vi "2_2_PatchCore_Inference(Camera).vi"() -> ()   [LabVIEW 2024]
uses:
  <vilib>/Ngene/DeepLTK Anomaly Detection Addon/DeepLTK_Anomaly_Detection_Addon/API/Controls/NN_Paths.ctl
  <vilib>/Ngene/Deep Learning Toolkit/Toolkit/NN_Data/API/NN_Dims(C,H,W).ctl
  <vilib>/Ngene/Deep Learning Toolkit/Toolkit/NN_Network/Controls/NN_Device.ctl
  subVIs/Visualizer/Controls/Display_Options.ctl
  subVIs/Visualizer/Controls/ROI_Display_Options.ctl
  subVIs/Visualizer/Controls/Heatmap_Display_Options.ctl
  subVIs/Visualizer/Controls/ColorMap.ctl
  <vilib>/Ngene/DeepLTK Anomaly Detection Addon/DeepLTK_Anomaly_Detection_Addon/API/Controls/MinMax.ctl
  subVIs/Camera/Controls/Camera_Settings.ctl
  <vilib>/Ngene/DeepLTK Anomaly Detection Addon/DeepLTK_Anomaly_Detection_Addon/API/Controls/NNPC_Setup.ctl
  <vilib>/vision/driver/IMAQdx.llb/IMAQdx Camera Control Mode.ctl
  <vilib>/vision/driver/IMAQdx.llb/IMAQdx Buffer Number Mode.ctl
  <vilib>/Ngene/DeepLTK Anomaly Detection Addon/DeepLTK_Anomaly_Detection_Addon/API/Controls/Feature_Scorer_Params.ctl
  <vilib>/Ngene/DeepLTK Anomaly Detection Addon/DeepLTK_Anomaly_Detection_Addon/API/Controls/Gaussian_Blur.ctl
  <vilib>/Ngene/DeepLTK Anomaly Detection Addon/DeepLTK_Anomaly_Detection_Addon/API/NNPC_Predict/NNPC_Predict(Single).vi
  <vilib>/Ngene/DeepLTK Anomaly Detection Addon/DeepLTK_Anomaly_Detection_Addon/DeepLTK_Anomaly_Detection_Addon.lvlib
  <vilib>/ptbypt/NI_PtbyPt.lvlib
  <vilib>/vision/driver/NI_Vision_Acquisition_Software.lvlib
  <vilib>/Ngene/Deep Learning Toolkit/Toolkit/Deep_Learning_Toolkit_by_Ngene.lvlib
  <vilib>/Ngene/CuLab - GPU Accelerated Toolkit/Toolkit/CuLab.lvlib
panel:
  in  "Tab Control":enum32{"Config", "Demo"}(tab)=enum."Demo"
  in  "Center_Crop_Size":i32=800
  in  "Device":T1
  in  "Trained_Model_Paths":T2={"CFG"=path "D:/Ngene/Projects_SVN/AD/Projects/2025/2025_04_09_VAD_RT_NIConnect/Models/NNPC_Cards_v2__25_04_09__17_01_43/NNPC_Cards_v2.cfg", "BIN"=path "D:/Ngene/Projects_SVN/AD/Projects/2025/2025_04_09_VAD_RT_NIConnect/Models/NNPC_Cards_v2__25_04_09__17_01_43/NNPC_Cards_v2.bin"}
  in  "Display_Options":T3={"ROI_Options"={"Color"=16711713, "Width"=4, "Drawing Mode"=enum."Frame"}, "Heatmap_Options"={"ColorMap"=enum."Jet", "Alpha"=0.4, "Heatmap Range"={"Min"=6.0, "Max"=-1.0}}, "Has GT?"=FALSE} {"Heatmap_Options"."Heatmap Range"."Min" format="%#_5g"}
  in  "Camera":refnum<k21>="cam5" caption="IMAQdx Session"
  in  "Rel Margin":sgl=0.02
  in  "Camera_Settings":T8={"Camera_Resolution"=270, "Focus"=17, "Exposure"=2, "Gain"=34, "WhiteB."=6457} {"WhiteB." min=2800 max=6500 step=1; "Gain" max=0; "Exposure" min=0 max=8 step=1; "Focus" max=0}
  out "Error Count":i16
  in  "Image_Thrshld":sgl=-1.0 format="%_5g"
  out "Pixel_Score(Max)":sgl=12.824394
  out "Img_Score":sgl=14.272138
  in  "Pixel_Thrshld":sgl=7.0 format="%_5g"
  out "Loop Time":dbl=0.692728653499671 format="%.2ps"
  out "Preproc. Time":dbl=0.014120406500296667 format="%.2ps"
  out "Dims_In":T9={"C"=3, "H"=256, "W"=256}
  in  "Stop":bool
  out "FPS":dbl=1.5954872600149606 format="%_3p"
  out "Inference Time":dbl=0.6267677749997347 format="%_3p"
  out "Device Name":string="sbRIO-9609"
  out "Prediction":bool=TRUE
  out "Anomaly Detection Results":T10(plugin-control)
  # "Unsupervised \nVisual Anomaly Detection"
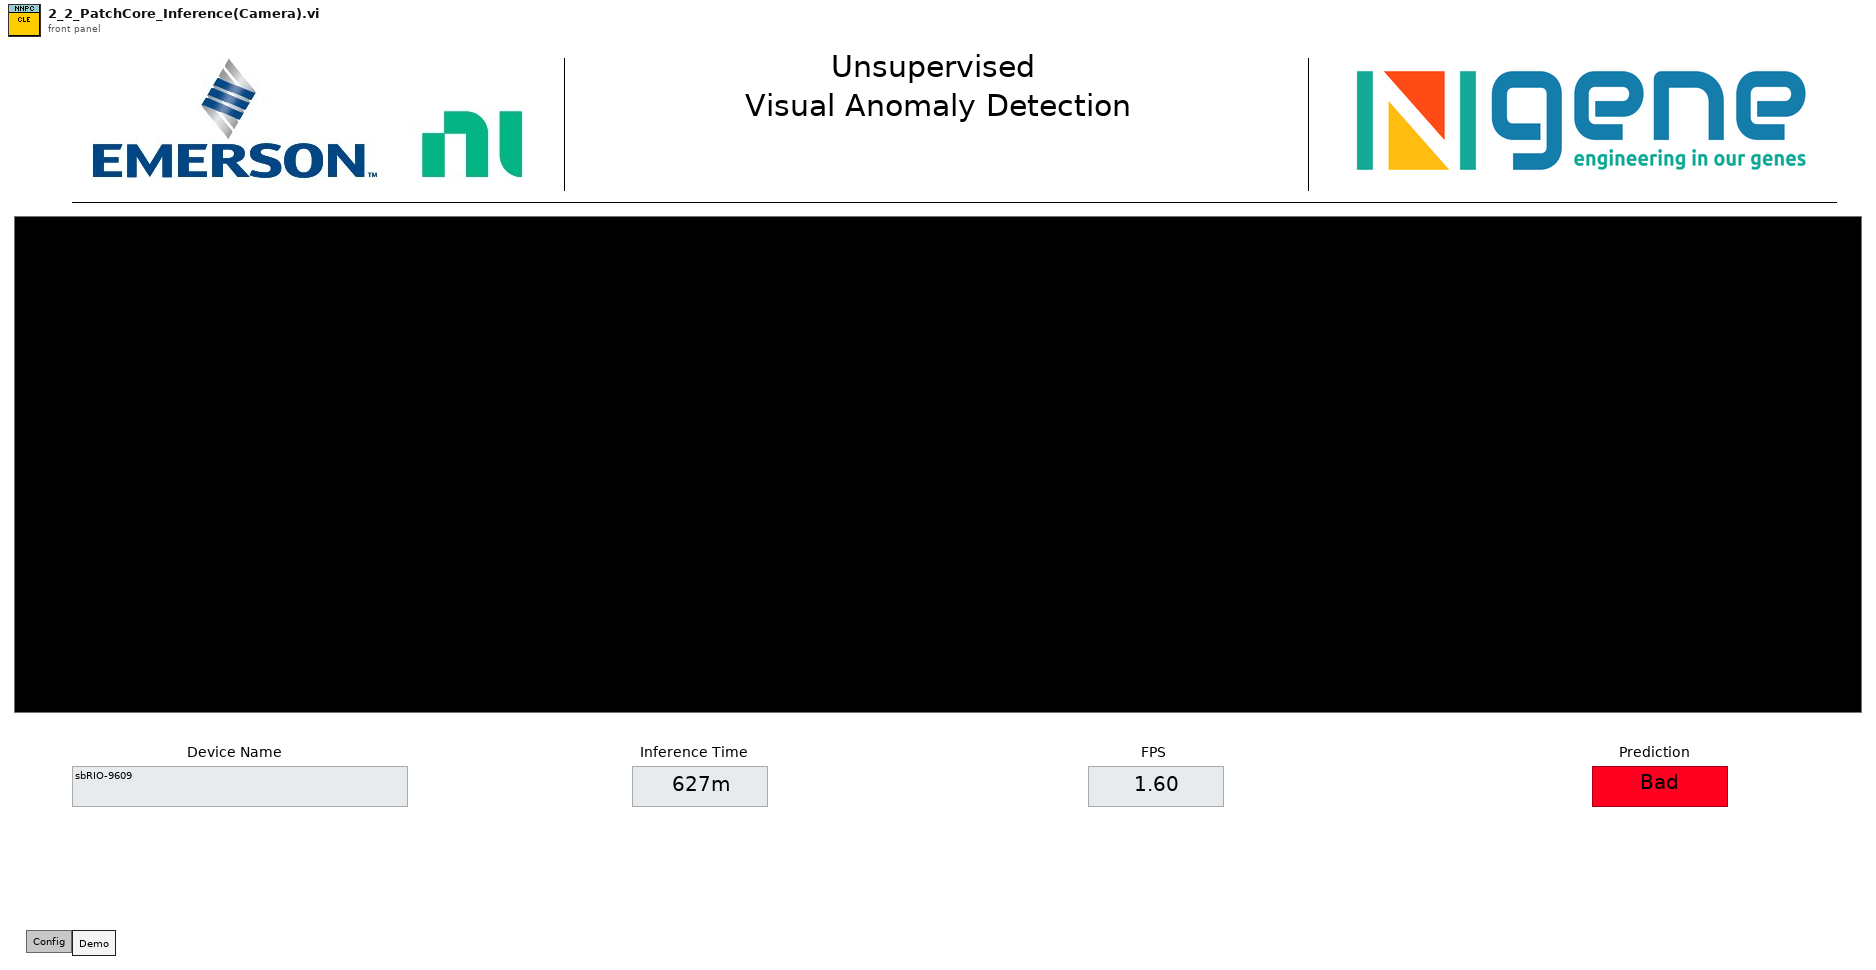
[diagram p1: front panel]
types:
  T1 = typedef "Deep_Learning_Toolkit_by_Ngene.lvlib/NN_Device.ctl" = enum16{"CPU", "GPU"}
  T2 = typedef "DeepLTK_Anomaly_Detection_Addon.lvlib/NN_Paths.ctl" = cluster{"CFG":path, "BIN":path}
  T3 = typedef "Display_Options.ctl" = cluster{"ROI_Options":T4, "Heatmap_Options":T5, "Has GT?":bool}
  T4 = typedef "ROI_Display_Options.ctl" = cluster{"Color":u32, "Width":u32, "Drawing Mode":enum16{"Frame", "Fill"}}
  T5 = typedef "Heatmap_Display_Options.ctl" = cluster{"ColorMap":T6, "Alpha":sgl, "Heatmap Range":T7}
  T6 = typedef "ColorMap.ctl" = enum16{"Jet", "Perula", "Inferno", "Plasma", "Viridis"}
  T7 = typedef "DeepLTK_Anomaly_Detection_Addon.lvlib/MinMax.ctl" = cluster{"Min":sgl, "Max":sgl}
  T8 = typedef "Camera_Settings.ctl" = cluster{"Camera_Resolution":i32, "Focus":u8, "Exposure":i32, "Gain":u32, "WhiteB.":i32}
  T9 = typedef "Deep_Learning_Toolkit_by_Ngene.lvlib/NN_Dims(C,H,W).ctl" = cluster{"C":i32, "H":i32, "W":i32}
  T10 = typedef "IMAQ Image.ctl" = refnum<image>
  T11 = typedef "Image Type" = u32
  T12 = typedef "NI_Vision_Acquisition_Software.lvlib/IMAQdx Camera Control Mode.ctl" = enum32{"Controller", "Listener"}
  T13 = typedef "DeepLTK_Anomaly_Detection_Addon.lvlib/NNPC_Setup.ctl" = cluster{"Input_Dims":T9, "mBatch":i32, "Device":T1, "GPU Id":i32}
  T14 = typedef "IMAQdx.ctl" = refnum<k21>
  T15 = typedef "DeepLTK_Anomaly_Detection_Addon.lvlib/NNPC_Evaluation_Results.ctl" = cluster{"Threshold(Image)":sgl, "Threshold(Pixel)":sgl, "Pixel_Range":cluster{"Min":sgl, "Max":sgl}}
  T16 = typedef "DeepLTK_Anomaly_Detection_Addon.lvlib/NNPC_PreProcessing_Options.ctl" = cluster{"DS_Name":string, "Input_Dims":T9, "Center Crop Size":i32, "Interpolation Type":u32, "Multi-Stage_DownSample?":bool, "Dataset_Stats":T17}
  T17 = typedef "DeepLTK_Anomaly_Detection_Addon.lvlib/NNPC_DS_Stats.ctl" = cluster{"means":T18, "stds":T18}
  T18 = typedef "DeepLTK_Anomaly_Detection_Addon.lvlib/Image_Stats_RGB.ctl" = cluster{"R":sgl, "G":sgl, "B":sgl}
  T19 = typedef "DeepLTK_Anomaly_Detection_Addon.lvlib/NNPC_Instance.ctl" = cluster{"NN out":T20, "MemBank_Data":T35, "Name":string}
  T20 = typedef "Deep_Learning_Toolkit_by_Ngene.lvlib/NN.ctl" = cluster{"Name":string, "No of Layers":i32, "mBatch":i32, "Layers":T21[], "Dimty":T22, "Dims_In":T9, "Dims_Out":T9, "Working_Dir":path, "Train?":bool, "Train_Params":T23, "LR_Update_Policy":T26, "Session Data":T28, "Ground_truth":T29, "NNg_hdls":T30, "NN_Device":T1, "GPU Id":i32, "Labels":string[], "Receptive Field":T31[], "Loss_Type":T32, "Loss_Cfg_Prms":variant, "NNG_WS":T33}
  T21 = typedef "Deep_Learning_Toolkit_by_Ngene.lvlib/NN_Layer_ref.ctl" = refnum<data-value>
  T22 = typedef "Deep_Learning_Toolkit_by_Ngene.lvlib/NN_In_Out_Dim-ty.ctl" = enum8{"In1D_Out1D", "In3D_Out1D", "In3D_Out3D", "In3D_OutBBox"}
  T23 = typedef "Deep_Learning_Toolkit_by_Ngene.lvlib/NN_Train_Params.ctl" = cluster{"Optimizer":T24, "Beta_1":sgl, "Beta_2":sgl, "Weight Decay(L1)":sgl, "Weight Decay(L2)":sgl, "Data_Sampling":T25}
  T24 = typedef "Deep_Learning_Toolkit_by_Ngene.lvlib/NN_Train_Optimizer.ctl" = enum16{"SGD", "Adam", "Adagrad", "Adadelta", "RMSProp", "Nesterov"}
  T25 = typedef "Deep_Learning_Toolkit_by_Ngene.lvlib/NN_Train_Data_Sampling.ctl" = enum16{"Random", "Sequential"}
  T26 = typedef "Deep_Learning_Toolkit_by_Ngene.lvlib/NN_LR_Policy_Cfg.ctl" = cluster{"Policy_Type":T27, "LR0":dbl, "k":sgl, "WarmUp_Policy":enum16{"Step", "Ramp"}, "WarmUp_Iter":i32, "WarmUp_Ratio":sgl}
  T27 = typedef "Deep_Learning_Toolkit_by_Ngene.lvlib/NN_LR_Policy_Type.ctl" = enum16{"Manual", "Step", "Exp", "1/t"}
  T28 = typedef "Deep_Learning_Toolkit_by_Ngene.lvlib/NN_Train_Session_Data.ctl" = cluster{"Epochs":sgl, "Tot_Iter":i32, "LR":sgl, "LR_iter":i32}
  T29 = typedef "Deep_Learning_Toolkit_by_Ngene.lvlib/NN_Ground_truth.ctl" = cluster{"Y":variant}
  T30 = typedef "Deep_Learning_Toolkit_by_Ngene.lvlib/nng_cuda_handles.ctl" = cluster{"cudnn":u64, "cublas":u64, "stream":u64, "curand":u64}
  T31 = typedef "Deep_Learning_Toolkit_by_Ngene.lvlib/NN_Dims(V,H).ctl" = cluster{"V":i32, "H":i32}
  T32 = typedef "Deep_Learning_Toolkit_by_Ngene.lvlib/NN_Loss_Type.ctl" = enum16{"None", "MSE", "CrossEntropy", "YOLO_v2", "YOLO_v4"}
  T33 = typedef "Deep_Learning_Toolkit_by_Ngene.lvlib/NNG_WS.ctl" = cluster{"NNG_WS_Mem":T34, "Max_WS_Size":i64}
  T34 = typedef "Deep_Learning_Toolkit_by_Ngene.lvlib/NNg_WS_Mem_DVR.ctl" = refnum<data-value>
  T35 = typedef "DeepLTK_Anomaly_Detection_Addon.lvlib/MemBank_and_Norm_Variants.ctl" = cluster{"MemBank":variant, "MemBank Norm":variant}
  T36 = typedef "DeepLTK_Anomaly_Detection_Addon.lvlib/Feature_Scorer_Params.ctl" = cluster{"Nearest_Neighbors":i32, "Calculate Anomaly Map":bool, "Gaussian_Blur":T37}
  T37 = typedef "DeepLTK_Anomaly_Detection_Addon.lvlib/Gaussian_Blur.ctl" = cluster{"Kernel_Size":i32, "Sigma":sgl}
  T38 = typedef "NI_Vision_Acquisition_Software.lvlib/IMAQdx Buffer Number Mode.ctl" = enum32{"Next", "Last", "Buffer Number", "Every", "Last New"}
  T39 = typedef "Anomaly_Detection_Results_Imgs.ctl" = cluster{"Image":T10, "Ground Truth":T10, "Predicted Heat Map":T10, "Predicted Mask":T10, "Segmentation":T10}
  T40 = typedef "CuLab.lvlib/Properties.ctl" = cluster{"Device ID":i32, "Name":string}
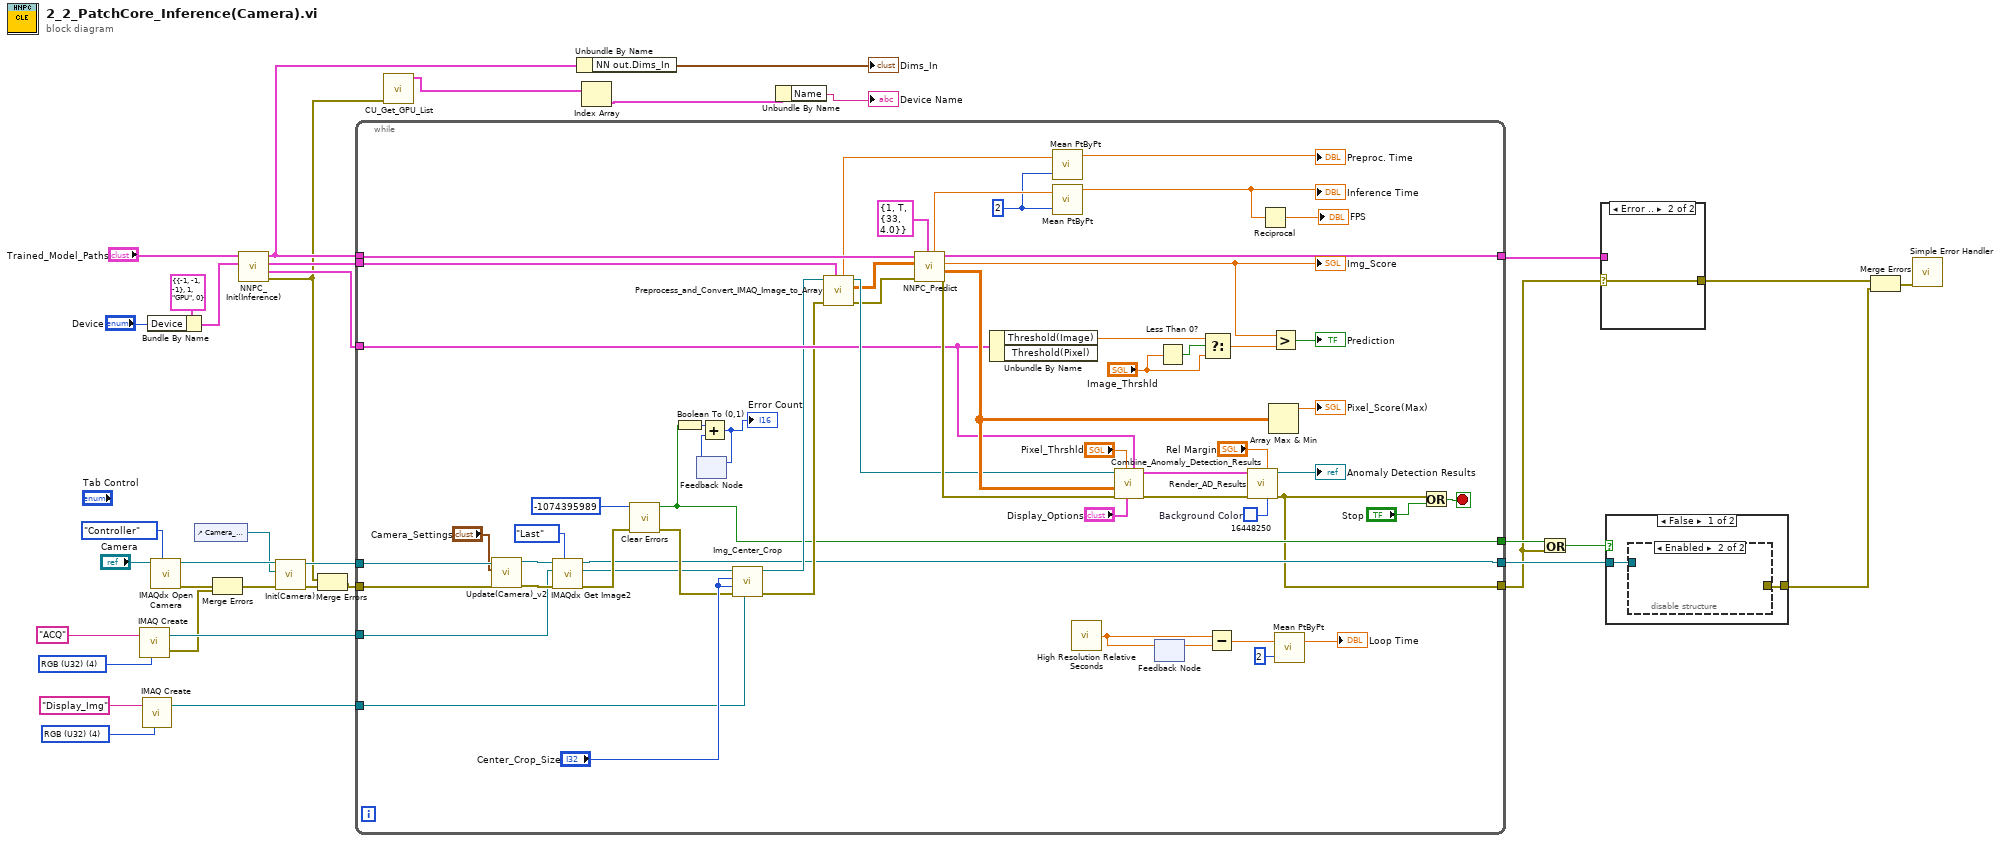
[diagram p0: block diagram]
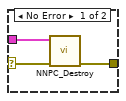
[diagram p2: hidden frame]
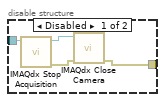
[diagram p3: hidden frame]
diagram:
  w10 = T11 4 items=["Grayscale (U8)", "Grayscale (I16)", "Grayscale (SGL)", "Complex (CSG)", "RGB (U32)", "HSL (U32)", "RGB (U64)", "Grayscale (U16)"] ("Image Type")
  w20 = T11 4 items=["Grayscale (U8)", "Grayscale (I16)", "Grayscale (SGL)", "Complex (CSG)", "RGB (U32)", "HSL (U32)", "RGB (U64)", "Grayscale (U16)"] ("Image Type")
  n1 = call "IMAQ Create"("Image Name"="ACQ", "Image Type"=w20) -> ("New Image"=w15:T10, "error out"=w12:errorcluster)  [unwired: 3 in]
  n2 = call "IMAQ Create"("Image Name"="Display_Img", "Image Type"=w10) -> ("New Image"=w8:T10)  [unwired: 3 in, 1 out]
  n3 = Bundle By Name(cluster=T13 {"Input_Dims"={"C"=-1, "H"=-1, "W"=-1}, "mBatch"=1, "Device"=enum."GPU", "GPU Id"=0} ("NNFE_CFG"), "Device"="Device") -> (w14:T13)
  n4 = call <vilib>:"IMAQdx Open Camera.vi"("Camera Control Mode"=IMAQdx_Camera_Control_Mode."Controller", "Session In"="Camera") -> ("error out"=w21:errorcluster, "Session Out"=w22:T14)  [unwired: 1 in, 7 out]
  n5 = control-ref of="Camera_Settings"() -> (w13:refnum<vi>)
  n6 = Merge Errors(w21, w12) -> (w18:errorcluster)
  n7 = call <vilib>:"NNPC_Init(Inference).vi"("NNPC_Setup"=w14, "NNPC_Paths"="Trained_Model_Paths") -> ("error out"=w4:errorcluster, "Evaluation_Results"=w32:T15, "PreProc_Options"=w33:T16, "NNPC_out"=w28:T19)  [unwired: 5 in, 1 out]
  n8 = call "Init(Camera).vi"("error in (no error)"=w18, "Camera_Settings_Ref"=w13, "Session in"=w22) -> ("error out"=w17:errorcluster, "Session out"=w16:T14)  [unwired: 7 in]
  n9 = Merge Errors(w4, w17) -> (w11:errorcluster)
  n10 = while {
    tunnel: w28 -> [w84]
    tunnel: [w79] -> w36
    tunnel: w33 -> [w71]
    tunnel: w32 -> [w66]
    tunnel: [w41] -> w31
    tunnel: [w40] -> w5
    tunnel: w11 -> [w59]
    tunnel: w16 -> [w62]
    tunnel: w15 -> [w58]
    tunnel: w8 -> [w48]
    tunnel: [w45] -> w7
    stop <- w78 stop-if-true
    w39 = 2 ("sample length")
    w77 = u32 16448250  # Background Color
    n11 = call "Update(Camera)_v2.vi"("error in (no error)"=w59, "Camera_Settings"="Camera_Settings", "Session in"=w62) -> ("error out"=w61:errorcluster, "Session out"=w60:T14)  [unwired: 7 in]
    n12 = call <vilib>:"IMAQdx Get Image2.vi"("Buffer Number Mode (Next)"=IMAQdx_Buffer_Number_Mode."Last", "error in"=w61, "Image In"=w58, "Session In"=w60) -> ("error out"=w50:errorcluster, "Image Out"=w49:T10, "Session Out"=w41:T14)  [unwired: 4 in, 1 out]
    n13 = call <vilib>:"Clear Errors.vi"("error in (no error)"=w50, "specific error code to clear (0: all)"=-1074395989) -> ("error out"=w52:errorcluster, "specific error cleared?"=w45:bool)  [unwired: 4 in]
    n14 = Boolean To (0,1)(Boolean=w45) -> (0, 1=w44:i16)
    n15 = feedback #1() -> (w46:i16)  [unwired: 1 in]
    n16 = Add(x=w44, y=w46) -> (x+y=w43:i16)
    "Error Count" <- w43
    n17 = feedback-in #1(w43) -> ()
    n18 = call "Img_Center_Crop.vi"("Image Dst"=w48, "error in (no error)"=w52, "height"="Center_Crop_Size", "width"="Center_Crop_Size", "Image In"=w49) -> ("error out"=w54:errorcluster, "Image Out"=w56:T10)  [unwired: 5 in]
    n19 = call "Preprocess_and_Convert_IMAQ_Image_to_Array.vi"("PreProcessing_Options"=w71, "error in (no error)"=w54, "Imaq Image In"=w56) -> ("error out"=w67:errorcluster, "Norm_Img_Out"=w53:sgl[][][], "Imaq Image Out"=w68:T10, "dT_Preprocessing"=w69:dbl)  [unwired: 5 in]
    n20 = call-poly <vilib>:"NNPC_Predict.vi"("Feature_Scorer_Params"=T36 {"Nearest_Neighbors"=1, "Calculate Anomaly Map"=TRUE, "Gaussian_Blur"={"Kernel_Size"=33, "Sigma"=4.0}}, "error in"=w67, "Image_in"=w53, "NNPC_in"=w84) -> ("error out"=w94:errorcluster, "Anomaly_Map"=w83:sgl[][], "Pred_Score"=w82:sgl, "NNPC_out"=w79:T19, "dT_Predict"=w76:dbl)  [unwired: 2 in, 1 out]
    "Img_Score" <- w82
    n21 = Unbundle By Name(w66) -> ("Threshold(Image)"=w75:sgl)  [unwired: 1 out]
    n22 = call <vilib>:"Mean PtByPt.vi"("x"=w69, "sample length"=w39) -> ("mean"=→"Preproc. Time":dbl)  [unwired: 2 in, 1 out]
    n23 = call <vilib>:"Mean PtByPt.vi"("x"=w76, "sample length"=w39) -> ("mean"=w38:dbl)  [unwired: 2 in, 1 out]
    "Inference Time" <- w38
    n24 = call <vilib>:"High Resolution Relative Seconds.vi"() -> ("relative seconds"=w73:dbl)
    n25 = call "Combine_Anomaly_Detection_Results.vi"("Evaluation_Results"=w66, "Display_Options"="Display_Options", "Pixel Anomaly Thrshld"="Pixel_Thrshld", "error in"=w94, "Anomaly Map"=w83, "Orig Image In"=w68) -> ("error out"=w93:errorcluster, "Anomaly Detection Rresults"=w92:T39)  [unwired: 3 in, 1 out]
    n26 = feedback #2() -> (w74:dbl)  [unwired: 1 in]
    n27 = feedback-in #2(w73) -> ()
    n28 = Less Than 0?(x="Image_Thrshld") -> (x < 0?=w88:bool)
    n29 = Select(t=w75, s=w88, f="Image_Thrshld") -> (s? t:f=w86:sgl)
    n30 = Subtract(x=w73, y=w74) -> (x-y=w72:dbl)
    n31 = call "Render_AD_Results.vi"("Background Color"=w77, "Rel._Margin"="Rel Margin", "error in"=w93, "Anomaly Detection Rresults"=w92) -> ("error out"=w40:errorcluster, "Anomaly Detection Results"=→"Anomaly Detection Results":T10)  [unwired: 6 in]
    n32 = Reciprocal(x=w38) -> (1/x=→"FPS":dbl)
    n33 = Array Max & Min(array=w83) -> (max value=→"Pixel_Score(Max)":sgl)  [unwired: 3 out]
    n34 = Greater?(x=w82, y=w86) -> (0:→"Prediction":bool)
    n35 = call <vilib>:"Mean PtByPt.vi"("x"=w72, "sample length"=2) -> ("mean"=→"Loop Time":dbl)  [unwired: 2 in, 1 out]
    n36 = Or(x=w40, y="Stop") -> (x .or. y?=w78:bool)
  }
  n37 = call <vilib>:"CU_Get_GPU_List.vi"("error in (no error)"=w4) -> ("Devices"=w3:T40[])  [unwired: 9 in, 1 out]
  n38 = Unbundle By Name(w28) -> ("NN out.Dims_In"=→"Dims_In":T9)
  n39 = Index Array(array=w3) -> (element=w2:T40)  [unwired: 1 in]
  n40 = Unbundle By Name(w2) -> ("Name"=→"Device Name":string)
  n41 = Or(x=w7, y=w5) -> (x .or. y?=w6:bool)
  n42 = case shown="Error .." w5 {
    selector: w5 -> [w95 w98]
    tunnel: w36 -> [w97 _]
    tunnel: [w96 w98] -> w35
    frame No Error {
      n43 = call <vilib>:"NNPC_Destroy.vi"("error in"=w95, "NNPC_in"=w97) -> ("error out"=w96:errorcluster)  [unwired: 9 in]
    }
    frame Error {
    }
  }
  n44 = case shown="False" w6 {
    tunnel: w31 -> [w100 _]
    tunnel: [w99 _] -> w29
    frame False {
      n45 = disable-structure shown="Enabled" {
        disable-tunnel: w100 -> [w104 _]
        disable-tunnel: [w101 _] -> w99
        frame Disabled {
          n46 = call <vilib>:"IMAQdx Stop Acquisition.vi"("Session In"=w104) -> ("error out"=w102:errorcluster, "Session Out"=w103:T14)  [unwired: 9 in]
          n47 = call <vilib>:"IMAQdx Close Camera.vi"("error in"=w102, "Session In"=w103) -> ("error out"=w101:errorcluster)  [unwired: 9 in]
        }
        frame Enabled {
        }
      }
    }
    frame True {
    }
  }
  n48 = Merge Errors(w35, w29) -> (w30:errorcluster)
  n49 = call <vilib>:"Simple Error Handler.vi"("error in (no error)"=w30) -> ()  [unwired: 4 in, 5 out]
